vi "Pololu-Set Position.vi"(4 "User Units Max":u16, 5 "Servo Units Max":u16, 6 "User Units Min":u16, 7 "Servo Units Min":u16, 8 "error in":errorcluster, 9 "Servo Chan":u16, 10 "position":u16(slide)=576 min=576 max=2416 scale=0.0..180.0, 11 "VISA resource name":refnum<visa-resource-name>) -> (0 "error out":errorcluster)   [LabVIEW 2018]
uses:
  Utils/Errors/Error.Error Code List.ctl
  <vilib>/Instr/_visa.llb/VISA Configure Serial Port (Instr).vi
panel:
  out "sent string":string
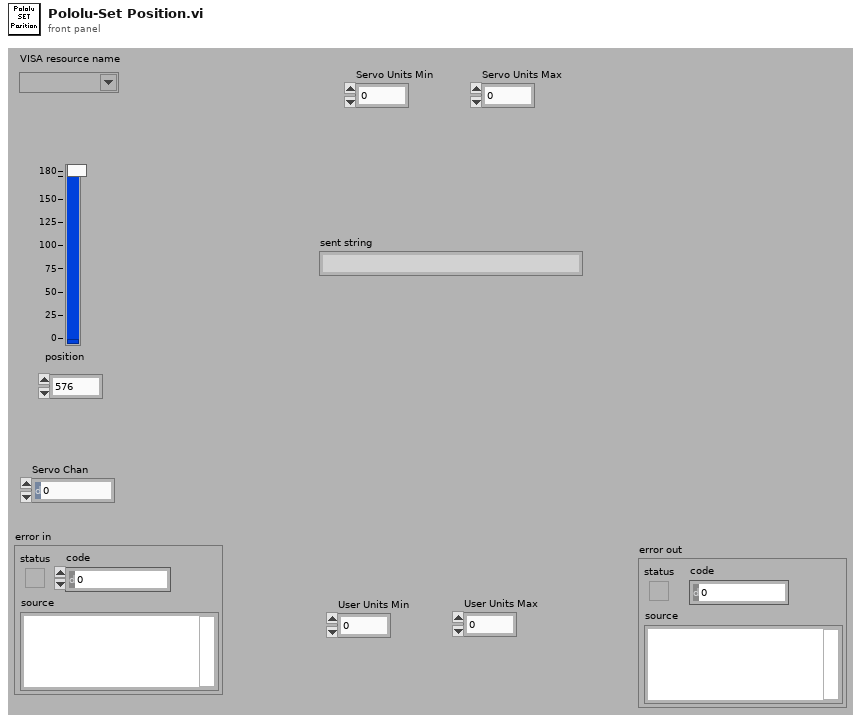
[diagram p1: front panel]
types:
  T1 = typedef "Error.Error Code List.ctl" = i32
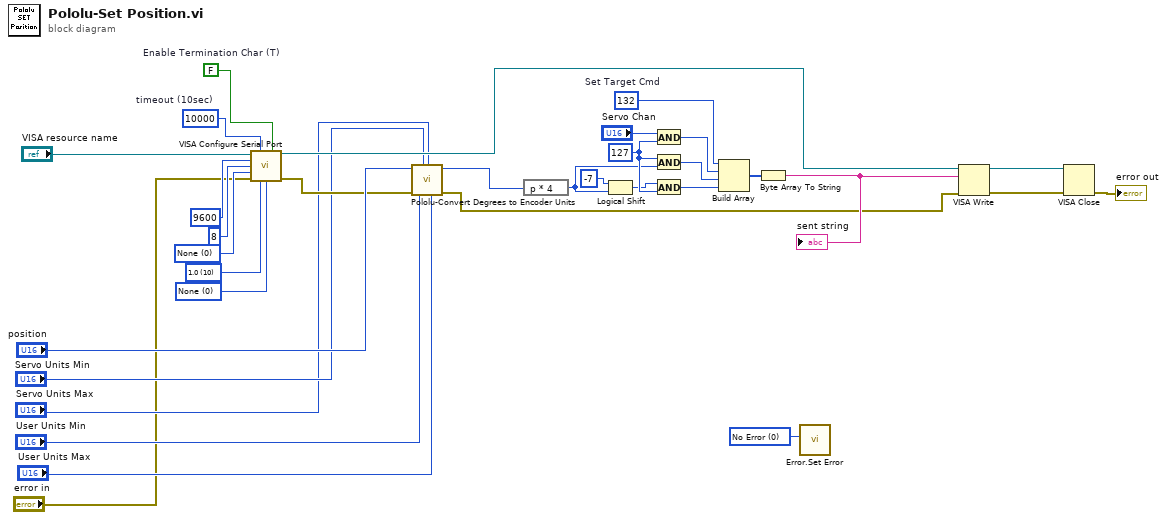
[diagram p0: block diagram]
diagram:
  w1 = T1 0 items=["No Error"=0, "Abort"=-2, "Misc"=-5000, "Fixture Error"=-5100, "File IO - General"=-5200, "FIle IO - Config Error"=-5201, "Instrument - General"=-5300, "Instrument - Serial Com"=-5301, "Instrument - Camera"=-5302, "Instrument - PS"=-5303, "Instrument - Oscilloscope"=-5304, "Instrument - Function Gen"=-5305, "Instrument - Load"=-5306, "Instrument - Meter"=-5307, "Instrument - Power Control"=-5308, "Instrument - Motion"=-5309, "Instrument - RF"=-5310, "System Exe"=-5400, "Image Processing"=-5500, "Communication"=-5600, "Script - Syntax Error"=-6000, "Script - Invalid Name or Param"=-6100, "Script - Timeout"=-6200, "Invalid Data"=-6300, "FW Update Error"=-6500] ("Std Code")
  w8 = u16 0 items=["None"=0, "XON/XOFF"=1, "RTS/CTS"=2, "DTR/DSR"=4] ("flow control")
  w9 = u16 10 items=["1.0"=10, "1.5"=15, "2.0"=20] ("stop bits")
  w10 = u16 0 items=["None", "Odd", "Even", "Mark", "Space"] ("parity")
  w13 = FALSE  # Enable Termination Char (T)
  w14 = u32 10000  # timeout (10sec)
  w23 = u8 132  # Set Target Cmd
  w25 = u8 127
  n1 = call-poly "VISA Configure Serial Port"("VISA resource name"="VISA resource name", "timeout (10sec)"=w14, "Enable Termination\nChar (T)"=w13, "baud rate (9600)"=u32 9600 ("baud rate"), "data bits (8)"=u16 8 ("data bits"), "parity (0:none)"=w10, "error in (no error)"="error in", "stop bits (10: 1 bit)"=w9, "flow control (0:none)"=w8) -> ("VISA resource name out"=w30:refnum<visa-resource-name>, "error out"=w16:errorcluster)  [unwired: 5 out]
  n2 = call "Pololu-Convert Degrees to Encoder Units.vi"("Deg Max"="User Units Max", "Encoder Units Max"="Servo Units Max", "Deg Min"="User Units Min", "Encoder Units Min"="Servo Units Min", "Error In"=w16, "Position Deg"="position") -> ("Error Out"=w15:errorcluster, "Position Encoder Units"=w17:u16)  [unwired: 4 in]
  n3 = expression code="p * 4"(w17) -> (w20:u16)
  n4 = Logical Shift(y=i8 -7, x=w20) -> (x << y=w22:u16)
  n5 = And(x="Servo Chan", y=w25) -> (x .and. y?=w26:u16)
  n6 = And(x=w25, y=w20) -> (x .and. y?=w27:u16)
  n7 = And(x=w22, y=w25) -> (x .and. y?=w28:u16)
  n8 = Build Array(w23, w26, w27, w28) -> (w18:u16[])
  n9 = Byte Array To String(unsigned byte array=w18) -> (string=w19:string)
  "sent string" <- w19
  n10 = call "Error.Set Error.vi"("Code"=w1) -> ()  [unwired: 6 in, 1 out]
  n11 = VISA Write(VISA resource name=w30, write buffer=w19, error in (no error)=w15) -> (VISA resource name out=w33:refnum<visa-resource-name>, error out=w32:errorcluster)  [unwired: 1 out]
  n12 = VISA Close(VISA resource name=w33, error in (no error)=w32) -> (error out=→"error out":errorcluster)
